vi "dispose engine.vi"(8 "error in":errorcluster, 11 "engine":u64) -> (0 "error out":errorcluster)   [LabVIEW 2016, in "async tls.lvlib"]
uses:
  async tls.lvlib
  lvasynctls.dll
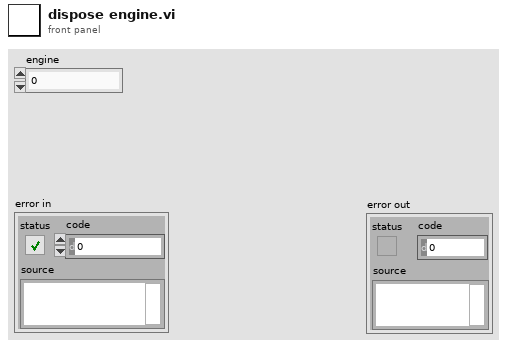
[diagram p1: front panel]
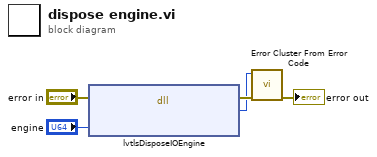
[diagram p0: block diagram]
diagram:
  n1 = dll-call lib="C:/Users/IEUser/Desktop/libasynclvtls/lvasynctls.dll" fn="lvtlsDisposeIOEngine"(error in="error in", "engine"="engine") -> (error out=w5:errorcluster, "err"=w4:i32)  [unwired: 3 in, 1 out]
  n2 = call <vilib>:"Error Cluster From Error Code.vi"("error in (no error)"=w5, "error code (0)"=w4) -> ("error out"=→"error out":errorcluster)  [unwired: 7 in]
